vi "New.vi"(11 "Number of samples (4)":i32) -> (0 "error out":errorcluster, 3 "Automatic Mode out":refnum<class "Automatic Mode.lvclass">)   [LabVIEW 2015, in "Automatic Mode.lvclass"]
uses:
  Automatic Mode.lvclass
  Automatic Mode.lvclass/Automatic Mode.ctl
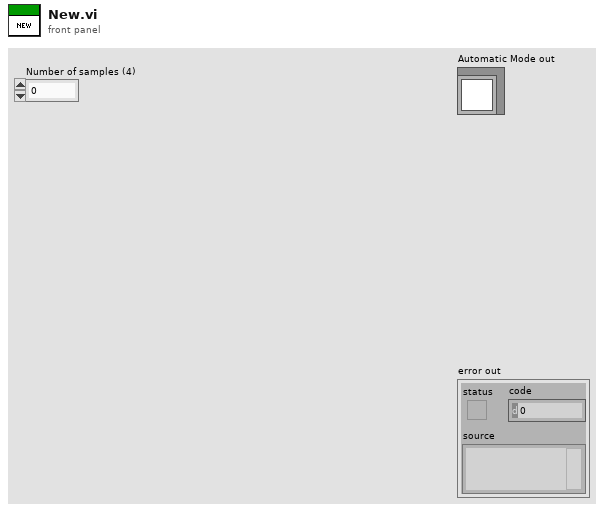
[diagram p1: front panel]
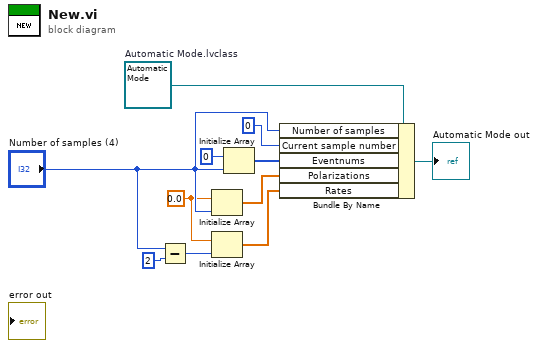
[diagram p0: block diagram]
diagram:
  w6 = 0.0 ("element")
  w11 = refnum<class "Automatic Mode.lvclass"> refnum  # Automatic Mode.lvclass
  n1 = Subtract(x="Number of samples (4)", y=2) -> (x-y=w9:i32)
  n2 = Initialize Array(w6, "Number of samples (4)") -> (w3:dbl[])
  n3 = Initialize Array(w6, w9) -> (w2:dbl[])
  n4 = Initialize Array(i64 0 ("element"), "Number of samples (4)") -> (w4:i64[])
  n5 = Bundle By Name(cluster=w11, "Number of samples"="Number of samples (4)", "Current sample number"=0, "Eventnums"=w4, "Polarizations"=w3, "Rates"=w2) -> (→"Automatic Mode out":refnum<class "Automatic Mode.lvclass">)
